vi "pad.vi"(8 "data length":i32, 11 "Last Block":u8[](array[numeric]) format="%02x") -> (2 "blocks":i32, 3 "Padding":u8[](array[numeric]) format="%02x")   [LabVIEW 2013, in "MD5.lvlib" / "MD5.lvclass"]
doc: "This VI creates a new string that represents the padding for the message string. The sum of the lengths of the message string and the padding string (in bytes) must be a multiple of 64."
uses:
  MD5.lvclass
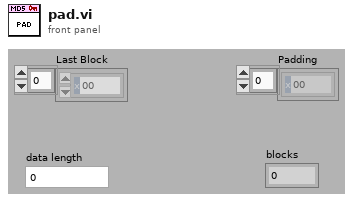
[diagram p1: front panel]
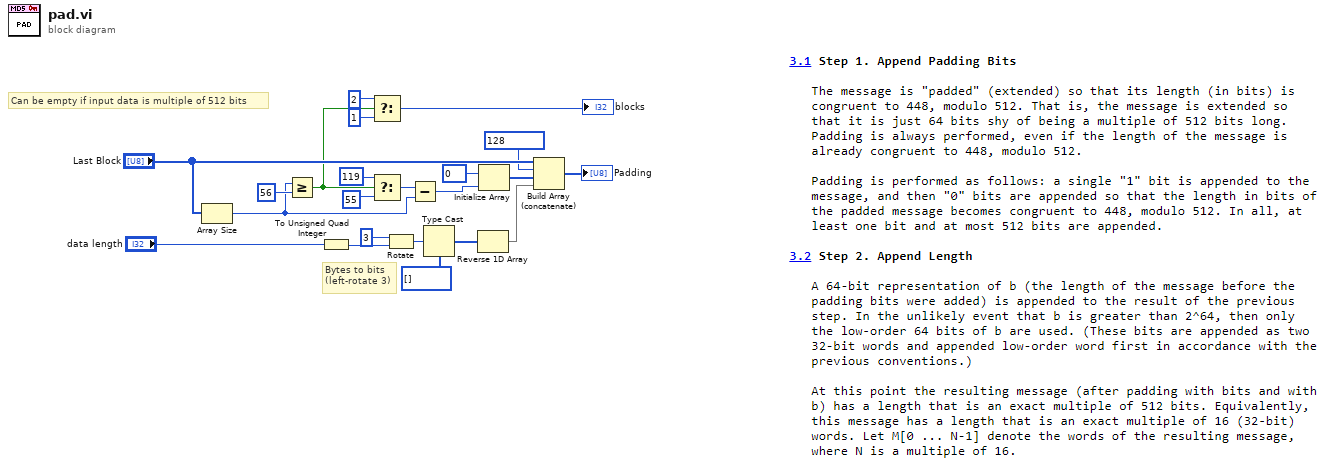
[diagram p0: block diagram]
diagram:
  # "Bytes to bits\n(left-rotate 3)"
  # "Can be empty if input data is multiple of 512 bits"
  n1 = Array Size(array="Last Block") -> (size(s)=w12:i32)
  n2 = Greater Or Equal?(x=w12, y=56) -> (x >= y?=w7:bool)
  n3 = To Unsigned Quad Integer(1:"data length") -> (0:w22:u64)
  n4 = Select(t=2 ("blocks"), s=w7, f=1 ("blocks")) -> (s? t:f=→"blocks":i32)
  n5 = Select(t=119 ("dimension size"), s=w7, f=55 ("dimension size")) -> (s? t:f=w11:i32)
  n6 = Rotate(1:w22, 2:i16 3 ("y")) -> (0:w19:u64)
  n7 = Subtract(x=w11, y=w12) -> (x-y=w10:i32)
  n8 = Type Cast(type=u8[] [] ("Last Block"), x=w19) -> (*(type *) &x=w3:u8[])
  n9 = Reverse 1D Array(array=w3) -> (reversed array=w2:u8[])
  n10 = Initialize Array(u8 0, w10) -> (w8:u8[])
  n11 = Build Array (concatenate)("Last Block", u8 128, w8, w2) -> (→"Padding":u8[])
